vi "Get Switches Status.vi"(10 "NewVal":bool[](array[boolean]), 11 "OldVal":bool[](array[boolean])) -> (3 "Zone Number - 1":i32)   [LabVIEW 2016]
doc: "Compare switch current status with the previous state. From this, Zone number is determined."
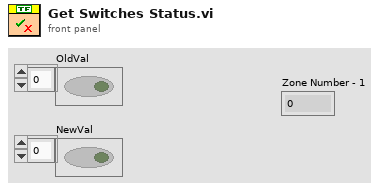
[diagram p1: front panel]
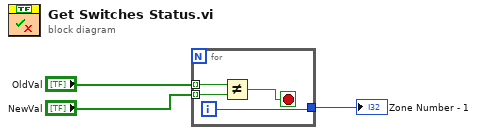
[diagram p0: block diagram]
diagram:
  n1 = for {
    tunnel: "OldVal" -> [w7] mode=indexing
    tunnel: "NewVal" -> [w6] mode=indexing
    tunnel: [w4] -> w3
    i -> [w4]
    stop <- w5 stop-if-true
    n2 = Not Equal?(x=w7, y=w6) -> (x != y?=w5:bool)
  }
  "Zone Number - 1" <- w3
